vi "ContinuousPressureAcquisition.vi"(8 "error in":errorcluster) -> (0 "error out":errorcluster)   [LabVIEW 2013]
uses:
  GlobalVariables/PressureAndTimeSamples.vi
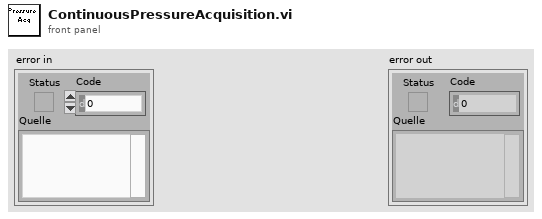
[diagram p1: front panel]
types:
  T1 = cluster{"TimeSamples":dbl[], "PressureSamples":dbl[]}
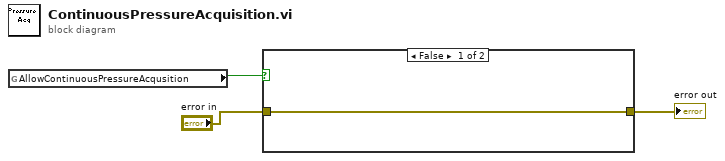
[diagram p0: block diagram]
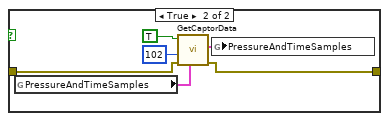
[diagram p2: hidden frame]
diagram:
  n1 = global read "AllowContinuousPressureAcquisition.vi" "AllowContinuousPressureAcqusition"() -> (w3:bool)
  n2 = case shown="False" w3 {
    tunnel: "error in" -> [w4 w6]
    tunnel: [w4 w5] -> w1
    frame False {
    }
    frame True {
      n3 = global read "PressureAndTimeSamples.vi" "PressureAndTimeSamples"() -> (w8:T1)
      n4 = call "GetCaptorData.vi"("Graph in"=w8, "error in"=w6, "Length"=102, "ON"=TRUE) -> ("error out"=w5:errorcluster, "Values"=w7:cluster{dbl[], dbl[]})  [unwired: 6 in]
      n5 = global write "PressureAndTimeSamples.vi" "PressureAndTimeSamples"(w7) -> ()
    }
  }
  "error out" <- w1
